vi "dBm_mW.vi"(11 "dBm":dbl) -> (3 "mW":dbl format="%#_13f")   [LabVIEW 2023]
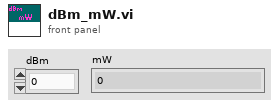
[diagram p1: front panel]
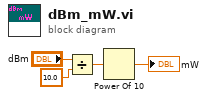
[diagram p0: block diagram]
diagram:
  n1 = Divide(x="dBm", y=10.0) -> (x/y=w2:dbl)
  n2 = Power Of 10(x=w2) -> (10^x=→"mW":dbl)
